vi "Pololu.Mgr - Set Speed.vi"(8 "error in (no error)":errorcluster, 9 "0.25us/10ms":dbl=10.0, 10 "Channel(use -1 for All)":i32=-1, 11 "PololuCtrl in":refnum<class "PololuCtrl.lvclass">) -> (0 "error out":errorcluster, 3 "PololuCtrl out":refnum<class "PololuCtrl.lvclass">)   [LabVIEW 2018, in "PololuCtrl.lvclass"]
uses:
  PololuCtrl.lvclass
  PololuCtrl.lvclass/PololuCtrl.ctl
  SubVIs/Pololu.Commands.ctl
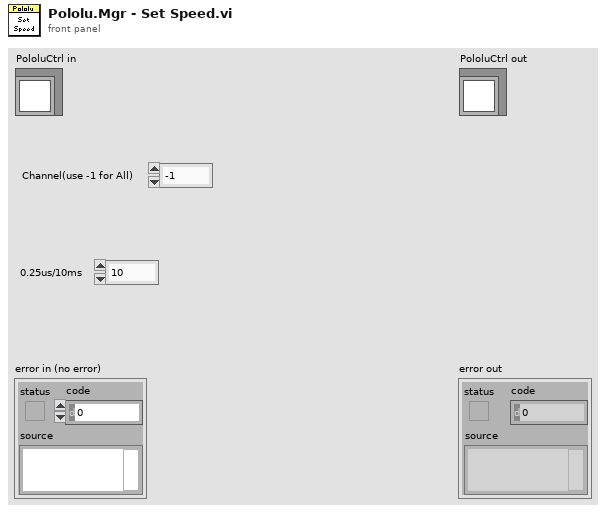
[diagram p1: front panel]
types:
  T1 = typedef "Pololu.Commands.ctl" = enum16{"Set Pos", "Set Speed", "Set Accel", "Get Pos", "Get Mov Status", "Get Errors"}
  T2 = typedef "Pololu.Device Config.ctl" = cluster{"Chan":u8, "Accel":u16, "Speed":u16, "Positions":dbl[], "Range Info":T3}
  T3 = typedef "Pololu.Device Range Config.ctl" = cluster{"Min us":dbl, "Max us":dbl, "Min deg":dbl, "Max deg":dbl, "LStopDeg":dbl, "UStopDeg":dbl}
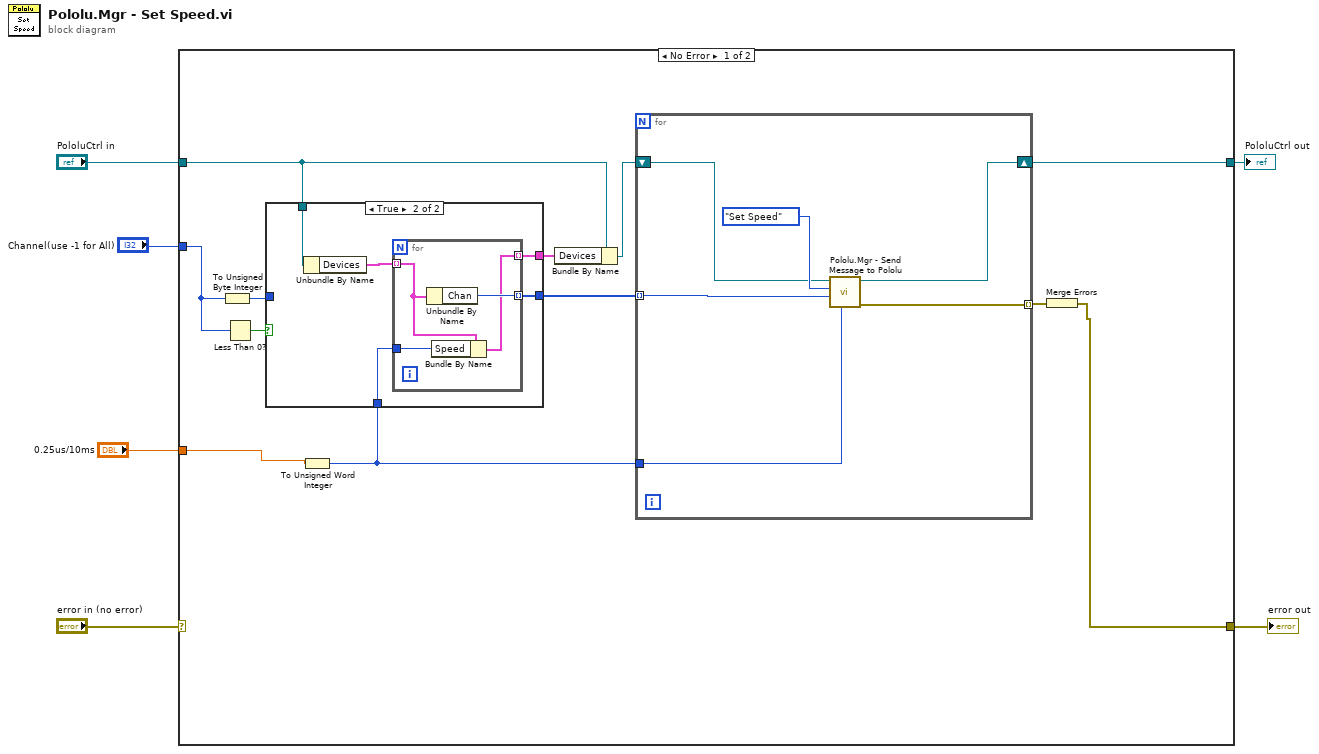
[diagram p0: block diagram]
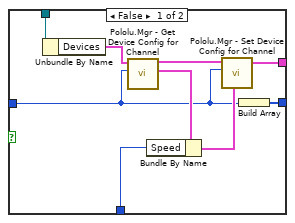
[diagram p2: hidden frame]
diagram:
  n1 = case shown="No Error" "error in (no error)" {
    selector: "error in (no error)" -> [_ w44]
    tunnel: [w15 w44] -> w5
    tunnel: [w17 w43] -> w3
    tunnel: "PololuCtrl in" -> [w10 w43]
    tunnel: "Channel(use -1 for All)" -> [w12 _]
    tunnel: "0.25us/10ms" -> [w7 _]
    frame No Error {
      n2 = To Unsigned Byte Integer(number=w12) -> (unsigned 8bit integer=w13:u8)
      n3 = Less Than 0?(x=w12) -> (x < 0?=w18:bool)
      n4 = To Unsigned Word Integer(number=w7) -> (unsigned 16bit integer=w8:u16)
      n5 = case shown="True" w18 {
        tunnel: w10 -> [w26 w32]
        tunnel: w13 -> [w20 _]
        tunnel: [w27 w31] -> w14
        tunnel: [w19 w29] -> w9
        tunnel: w8 -> [w23 w28]
        frame False {
          n6 = Unbundle By Name(w26) -> ("Devices"=w25:T2[])
          n7 = call "Pololu.Mgr - Get Device Config for Channel.vi"("Channel"=w20, "Devices"=w25) -> ("Device"=w24:T2, "Devices Out"=w22:T2[])  [unwired: 7 in, 1 out]
          n8 = Bundle By Name(cluster=w24, "Speed"=w23) -> (w21:T2)
          n9 = call "Pololu.Mgr - Set Device Config for Channel.vi"("Device"=w21, "Channel"=w20, "Devices"=w22) -> ("Devices Out"=w19:T2[])  [unwired: 7 in, 1 out]
          n10 = Build Array(w20) -> (w27:u8[])
        }
        frame True {
          n11 = Unbundle By Name(w32) -> ("Devices"=w30:T2[])
          n12 = for {
            tunnel: w30 -> [w35] mode=indexing
            tunnel: [w36] -> w31 mode=indexing
            tunnel: [w34] -> w29 mode=indexing
            tunnel: w28 -> [w33]
            n13 = Unbundle By Name(w35) -> ("Chan"=w36:u8)
            n14 = Bundle By Name(cluster=w35, "Speed"=w33) -> (w34:T2)
          }
        }
      }
      n15 = Bundle By Name(cluster=w10, "Devices"=w9) -> (w11:refnum<class "PololuCtrl.lvclass">)
      n16 = for {
        tunnel: w8 -> [w39]
        shift-right: [w41] -> w17
        shift-left: w11 -> [w37]
        tunnel: [w40] -> w16 mode=indexing
        tunnel: w14 -> [w38] mode=indexing
        n17 = call "Pololu.Mgr - Send Message to Pololu.vi"("Value"=w39, "Channel"=w38, "Command"=Pololu.Commands."Set Speed", "PololuCtrl in"=w37) -> ("error out"=w40:errorcluster, "PololuCtrl out"=w41:refnum<class "PololuCtrl.lvclass">)  [unwired: 5 in, 1 out]
      }
      n18 = Merge Errors(w16) -> (w15:errorcluster)
    }
    frame Error {
    }
  }
  "error out" <- w5
  "PololuCtrl out" <- w3
